vi "Climber.vi"() -> ()   [LabVIEW 2019]
uses:
  <vilib>/Rock Robotics/WPI/Utilities/WPI_GetSetVariantRefNum.vi
panel:
  in  "Winch speed":dbl(slide) scale=0.0..1.0
  in  "Simulate Stop":bool
  in  "Simulate Bottom Switch":bool
  in  "Simulate Top Switch":bool
  in  "Simulate Up Button":bool
  in  "Simulate Down Button":bool
  out "Climber Motor Output":dbl
  in  "Trolly speed":dbl(slide) scale=0.0..100.0
  in  "Down Speed":dbl=0.2
  in  "Up Speed":dbl=0.2
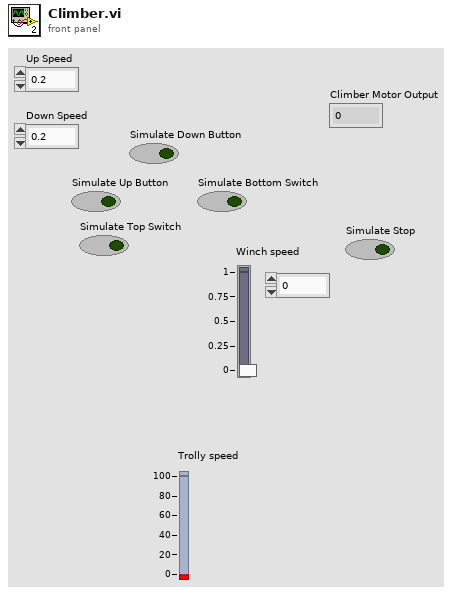
[diagram p1: front panel]
types:
  T1 = typedef "WPI_SwitchDevRef.ctl" = cluster{"DevStatus":errorcluster, "DIO Channel":T2, "CntIndex":T3, "Normally Closed":bool}
  T2 = typedef "FPGA_DIOChannel.ctl" = enum8{"DIO 0", "DIO 1", "DIO 2", "DIO 3", "DIO 4", "DIO 5", "DIO 6", "DIO 7", "DIO 8", "DIO 9", "DIO MXP 0", "DIO MXP 1", "DIO MXP 2", "DIO MXP 3", "DIO MXP 4", "DIO MXP 5", "DIO MXP 6", "DIO MXP 7", "DIO MXP 8", "DIO MXP 9", "DIO MXP 10", "DIO MXP 11", "DIO MXP 12", "DIO MXP 13", "DIO MXP 14", "DIO MXP 15", "SPI Port CS1", "SPI Port CS2", "SPI Port CS3", "SPI Port MISO", "SPI Port MOSI", "Invalid"}
  T3 = typedef "FPGA_CounterCtrSystemIndex.ctl" = enum8{"Ctr 0", "Ctr 1", "Ctr 2", "Ctr 3", "Ctr 4", "Ctr 5", "Ctr 6", "Ctr 7", "Invalid"}
  T4 = typedef "WPI_JoystickDevRef.ctl" = cluster{"Device":T5}
  T5 = typedef "WPI_JoystickDeviceEnum.ctl" = enum16{"USB 0", "USB 1", "USB 2", "USB 3", "USB 4", "USB 5"}
  T6 = typedef "WPI_MotorControlDeviceRef.ctl" = cluster{"DeviceStatus":errorcluster, "Type":T7, "PWM":cluster{"PWM Channel":T8, "DeadBand":T9}, "CAN":cluster{"Device Number":u8, "SetOutput VI Ref":variant, "GetOutput VI Ref":variant, "Enable VI Ref":variant, "Disable VI Ref":variant, "Data":variant}, "Invert":bool, "DIO PWM":cluster{"PWM \"Enable\" Channel":T8, "DIOChannel":T2, "PWM Rate":dbl}}
  T7 = typedef "WPI_MotorControlType.ctl" = enum16{"PWM", "CAN", "DIO PWM"}
  T8 = typedef "FPGA_DIOPWMChannel.ctl" = enum8{"PWM 0", "PWM 1", "PWM 2", "PWM 3", "PWM 4", "PWM 5", "PWM 6", "PWM 7", "PWM 8", "PWM 9", "PWM MXP 0", "PWM MXP 1", "PWM MXP 2", "PWM MXP 3", "PWM MXP 4", "PWM MXP 5", "PWM MXP 6", "PWM MXP 7", "PWM MXP 8", "PWM MXP 9", "Invalid"}
  T9 = typedef "WPI_PWMDeadband.ctl" = cluster{"Name":string, "maxPositivePwm":i32, "minPositivePwm":i32, "centerPwm":i32, "maxNegativePwm":i32, "minNegativePwm":i32, "angularRange":u16}
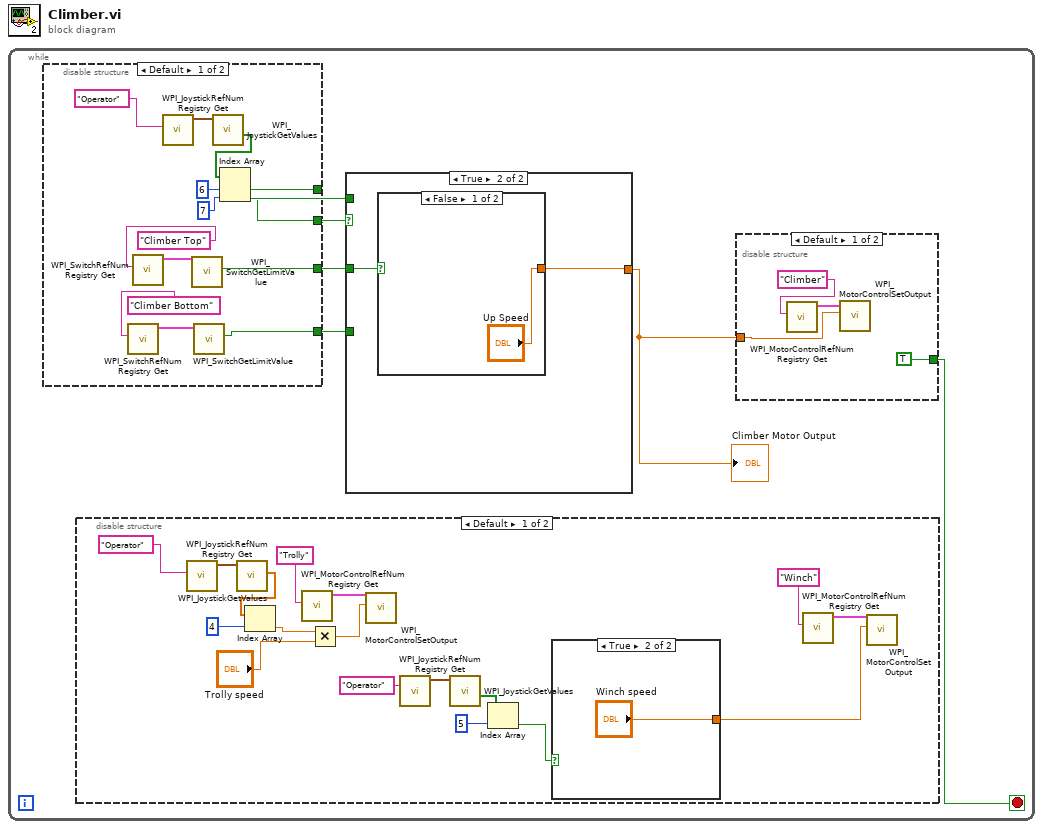
[diagram p0: block diagram]
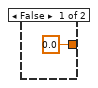
[diagram p2: hidden frame]
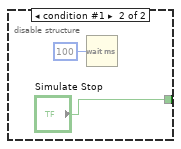
[diagram p4: hidden frame]
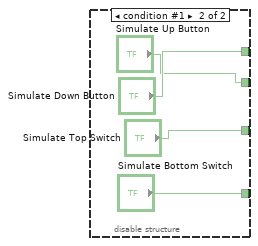
[diagram p5: hidden frame]
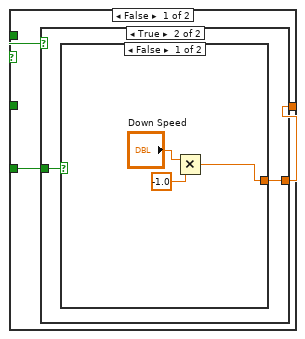
[diagram p6: hidden frame]
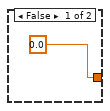
[diagram p7: hidden frame]
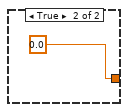
[diagram p8: hidden frame]
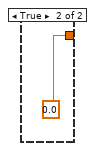
[diagram p9: hidden frame]
diagram:
  n1 = while {
    stop <- w1 stop-if-true
    n2 = disable-structure shown="Default" {
      disable-tunnel: [w37 "Simulate Up Button"] -> w2
      disable-tunnel: [w41 "Simulate Bottom Switch"] -> w4
      disable-tunnel: [w38 "Simulate Down Button"] -> w3
      disable-tunnel: [w44 "Simulate Top Switch"] -> w5
      frame condition #0 (active) {
        n3 = call <vilib>:"WPI_SwitchRefNum Registry Get.vi"("refnum name"="Climber Bottom") -> ("SwitchDevRef"=w40:T1)  [unwired: 9 in, 1 out]
        n4 = call <vilib>:"WPI_SwitchRefNum Registry Get.vi"("refnum name"="Climber Top") -> ("SwitchDevRef"=w43:T1)  [unwired: 9 in, 1 out]
        n5 = call <vilib>:"WPI_JoystickRefNum Registry Get.vi"("refnum name"="Operator") -> ("JoystickDevRef"=w35:T4)  [unwired: 1 in, 9 out]
        n6 = call <vilib>:"WPI_SwitchGetLimitValue.vi"("SwitchDevRef"=w43) -> ("Switch Pressed"=w44:bool)  [unwired: 8 in, 2 out]
        n7 = call <vilib>:"WPI_SwitchGetLimitValue.vi"("SwitchDevRef"=w40) -> ("Switch Pressed"=w41:bool)  [unwired: 8 in, 2 out]
        n8 = call <vilib>:"WPI_JoystickGetValues.vi"("JoystickDevRef"=w35) -> ("Buttons"=w36:bool[])  [unwired: 6 in, 4 out]
        n9 = Index Array(array=w36, index #1=6 ("index"), index #2=7 ("index")) -> (element #1=w38:bool, element #2=w37:bool)
      }
      frame condition #1 {
      }
    }
    n10 = disable-structure shown="Default" {
      frame condition #0 (active) {
        n11 = call <vilib>:"WPI_JoystickRefNum Registry Get.vi"("refnum name"="Operator") -> ("JoystickDevRef"=w21:T4)  [unwired: 1 in, 9 out]
        n12 = call <vilib>:"WPI_JoystickGetValues.vi"("JoystickDevRef"=w21) -> ("Axes"=w20:dbl[])  [unwired: 6 in, 4 out]
        n13 = Index Array(array=w20, index=4) -> (element=w19:dbl)
        n14 = call <vilib>:"WPI_MotorControlRefNum Registry Get.vi"("refnum name"="Trolly") -> ("MotorControlDevRef"=w23:T6)  [unwired: 9 in, 1 out]
        n15 = Multiply(x=w19, y="Trolly speed") -> (x*y=w18:dbl)
        n16 = call <vilib>:"WPI_MotorControlSetOutput.vi"("Output"=w18, "MotorControlDevRef"=w23) -> ()  [unwired: 7 in, 3 out]
        n17 = call <vilib>:"WPI_JoystickRefNum Registry Get.vi"("refnum name"="Operator") -> ("JoystickDevRef"=w12:T4)  [unwired: 1 in, 9 out]
        n18 = call <vilib>:"WPI_JoystickGetValues.vi"("JoystickDevRef"=w12) -> ("Buttons"=w10:bool[])  [unwired: 6 in, 4 out]
        n19 = Index Array(array=w10, index=5) -> (element=w13:bool)
        n20 = case shown="True" w13 {
          tunnel: [0.0 ("Winch speed") "Winch speed"] -> w7
          frame False {
          }
          frame True {
          }
        }
        n21 = call <vilib>:"WPI_MotorControlRefNum Registry Get.vi"("refnum name"="Winch") -> ("MotorControlDevRef"=w9:T6)  [unwired: 9 in, 1 out]
        n22 = call <vilib>:"WPI_MotorControlSetOutput.vi"("Output"=w7, "MotorControlDevRef"=w9) -> ()  [unwired: 7 in, 3 out]
      }
      frame condition #1 {
      }
    }
    n23 = case shown="True" w2 {
      tunnel: w3 -> [w49 _]
      tunnel: [w51 w60] -> w6
      tunnel: w4 -> [w50 _]
      tunnel: w5 -> [_ w59]
      frame False {
        n24 = case shown="True" w49 {
          tunnel: [0.0 ("Up Speed") w53] -> w51
          tunnel: w50 -> [_ w54]
          frame False {
          }
          frame True {
            n25 = case shown="False" w54 {
              tunnel: [w57 0.0 ("Up Speed")] -> w53
              frame False {
                n26 = Multiply(x="Down Speed", y=-1.0) -> (x*y=w57:dbl)
              }
              frame True {
              }
            }
          }
        }
      }
      frame True {
        n27 = case shown="False" w59 {
          tunnel: ["Up Speed" 0.0 ("Up Speed")] -> w60
          frame False {
          }
          frame True {
          }
        }
      }
    }
    "Climber Motor Output" <- w6
    n28 = disable-structure shown="Default" {
      disable-tunnel: w6 -> [w28 _]
      disable-tunnel: [TRUE "Simulate Stop"] -> w1
      frame condition #0 (active) {
        n29 = call <vilib>:"WPI_MotorControlRefNum Registry Get.vi"("refnum name"="Climber") -> ("MotorControlDevRef"=w27:T6)  [unwired: 9 in, 1 out]
        n30 = call <vilib>:"WPI_MotorControlSetOutput.vi"("Output"=w28, "MotorControlDevRef"=w27) -> ()  [unwired: 7 in, 3 out]
      }
      frame condition #1 {
        n31 = Wait (ms)(milliseconds to wait=u32 100) -> ()  [unwired: 1 out]
      }
    }
  }
